vi "Experiment header-Get typedef cluster ref.vi"(8 "error in (no error)":errorcluster, 11 "Header file type":T12) -> (0 "error out":errorcluster, 3 "Header prameter control refs[]":refnum<vi>[](array[refnum]))   [LabVIEW 2013]
uses:
  Typedefs/Header params-Funct acq w rectangles.ctl
  Typedefs/Frame Size.ctl
  Typedefs/Header parameters cluster-Zstack.ctl
  Typedefs/Header parameters cluster-Live imaging.ctl
  Typedefs/AOL modes.ctl
  Typedefs/Plane Mode.ctl
  Typedefs/Header parameters cluster-ALL.ctl
  Typedefs/Imaging Protocols enum.ctl
  Typedefs/Objective selector control enum.ctl
  Typedefs/Header file type enum.ctl
  Typedefs/Controls/AOL_Globals.ctl
panel:
  in  "Parameters tab":T1(tab)
  in  "All header parameters":T2={"Imaging Protocol"=enum."AOL Z-Stack", "Number of POI"=0, "Number of Miniscans"=0, "Number of Trials"=0, "Number of Cycles "=0, "# Averaged Frames"=0, "Laser power (%)"=0, "Pockels"=0.0, "Acquisition Length (sec)"=0.0, "Fill time (us)"=0.0, "POI Dwell time (us)"=0.0, "Miniscan Dwell time per pixel (us)"=0.0, "PMT 1"=0.0, "PMT 2"=0.0, "Back Apperture"=0.0, "Zoom"=0.0, "Frame Size"=0, "Center Frequency"=0.0, "Field of View"=0.0, "DwellTime (us)"=0.0, "Wavelength (nm)"=0.0, "AOL Z"=0.0, "AOL Mode"=enum."Raster", "GridXY"=0.0, "GridZ"=0.0, "TriggerDelay (sec)"=0.0, "Number of Pixels in Miniscan"=0, "Experiment folder path"=path "", "X centre"=0.0, "Y centre"=0.0, "Angle (degrees)"=0.0, "Plane Mode"=0, "Software version"=0.0, "Objective"="Olympus  20X", "MotorZ Calibration"=0, "Pockels Calibration"=0, "Threshold"=[], "Video length (sec)"=0.0, "Frame rate (fps)"=0, "Rectangle ROI length (pixels)"=0, "Rectangle ROI height (pixels)"=0} {"Pockels" format="%#.6g"; "Software version" format="%#.6g"; "Plane Mode" items=["XY Plane"]; "Angle (degrees)" format="%#.6g"; "Frame Size" items=["100X100"=100, "128X128"=128, "200X200"=200, "256X256"=256, "512X512"=512, "1024x1024"=1024, "2048x2048"=2048]; "Back Apperture" format="%#.6g"; "PMT 2" format="%#.6g"; "PMT 1" format="%#.6g"; "Miniscan Dwell time per pixel (us)" format="%#.6g"; "Zoom" format="%#.6g"; "POI Dwell time (us)" format="%#.6g"; "Acquisition Length (sec)" format="%#.6g"; "Fill time (us)" format="%#.6g"}
  in  "Header parameters-Zstack":T8={"Number of POI"=0, "Number of Miniscans"=0, "Number of Trials"=0, "Number of Cycles "=0, "# Averaged Frames"=0, "Laser power (%)"=0, "Pockels"=0.0, "Acquisition Length (sec)"=0.0, "Fill time (us)"=0.0, "DwellTime (us)"=0.0, "Miniscan Dwell time per pixel (us)"=0.0, "PMT 1"=0.0, "PMT 2"=0.0, "Back Apperture"=0.0, "Zoom"=0.0, "Number of Pixels in Miniscan"=0, "Frame Size"=200, "Field of View"=0.0, "X centre"=0.0, "Y centre"=0.0, "AOL Z"=0.0} {"Frame Size" items=["100X100"=100, "128X128"=128, "200X200"=200, "256X256"=256, "512X512"=512, "1024x1024"=1024, "2048x2048"=2048]; "Back Apperture" format="%#.6g"; "Pockels" format="%#.6g"; "PMT 2" format="%#.6g"; "PMT 1" format="%#.6g"; "Miniscan Dwell time per pixel (us)" format="%#.6g"; "Zoom" format="%#.6g"; "DwellTime (us)" format="%#.6g"; "Acquisition Length (sec)" format="%#.6g"; "Fill time (us)" format="%#.6g"}
  in  "Header params-Funct acq w rectangles":T9={"Number of POI"=0, "Number of Miniscans"=0, "Number of Trials"=0, "Number of Cycles "=0, "# Averaged Frames"=0, "Laser power (%)"=0, "Pockels"=0.0, "Acquisition Length (sec)"=0.0, "Fill time (us)"=0.0, "DwellTime (us)"=0.0, "Miniscan Dwell time per pixel (us)"=0.0, "PMT 1"=0.0, "PMT 2"=0.0, "Back Apperture"=0.0, "Zoom"=0.0, "Number of Pixels in Miniscan"=0, "Frame Size"=200, "Field of View"=0.0, "X centre"=0.0, "Y centre"=0.0, "AOL Z"=0.0, "Rectangle ROI length (pixels)"=0, "Rectangle ROI height (pixels)"=0} {"Frame Size" items=["100X100"=100, "128X128"=128, "200X200"=200, "256X256"=256, "512X512"=512, "1024x1024"=1024, "2048x2048"=2048]; "Back Apperture" format="%#.6g"; "Pockels" format="%#.6g"; "PMT 2" format="%#.6g"; "PMT 1" format="%#.6g"; "Miniscan Dwell time per pixel (us)" format="%#.6g"; "Zoom" format="%#.6g"; "DwellTime (us)" format="%#.6g"; "Acquisition Length (sec)" format="%#.6g"; "Fill time (us)" format="%#.6g"}
  in  "Header parameters-Live imaging":T10={"Frame Size"=200, "Field of View"=0.0, "Zoom"=0, "X centre"=0.0, "Y centre"=0.0, "DwellTime (us)"=0.0, "AOL Z"=0.0, "Wavelength (nm)"=0.0, "Laser power (%)"=0, "Pockels"=0.0, "Back Apperture"=0.0, "PMT 1"=0.0, "PMT 2"=0.0, "# Averaged Frames"=0, "AOL Mode"=enum."Raster", "Angle (degrees)"=0.0, "Plane Mode"=0, "Video length (sec)"=0.0, "Frame rate (fps)"=0, "Fill time (us)"=0.0} {"Fill time (us)" format="%#.6g"; "Back Apperture" format="%#.6g"; "Pockels" format="%#.6g"; "Plane Mode" items=["XY Plane"]; "Angle (degrees)" format="%#.6g"; "Frame Size" items=["100X100"=100, "128X128"=128, "200X200"=200, "256X256"=256, "512X512"=512, "1024x1024"=1024, "2048x2048"=2048]; "PMT 2" format="%#.6g"; "PMT 1" format="%#.6g"}
  in  "AOL_Globals":T11={"Imaging Protocol"=enum."AOL Z-Stack", "Number of POI"=0, "Number of Miniscans"=0, "Number of Trials"=0, "Number of Cycles "=0, "# Averaged Frames"=0, "Laser power (%)"=0, "Pockels"=0.0, "Acquisition Length (sec)"=0.0, "Fill time (us)"=0.0, "POI Dwell time (us)"=0.0, "Miniscan Dwell time per pixel (us)"=0.0, "PMT 1"=0.0, "PMT 2"=0.0, "Back Apperture"=200.0, "Frame Size"=0, "Center Frequency"=0.0, "Field of View"=0.0, "DwellTime (us)"=0.0, "Wavelength (nm)"=0.0, "Zoom"=0.0, "AOL Z"=0.0, "AOL Mode"=enum."Raster", "GridXY"=0.0, "GridZ"=0.0, "TriggerPeriod (sec)"=0.0, "Number of Pixels in Miniscan"=0, "Experiment folder path"=path "", "X centre"=0.0, "Y centre"=0.0, "Angle (degrees)"=0.0, "Plane Mode"=0, "Threshold"=[], "Regenerate Chirps"=FALSE, "Rectangle ROI length (pixels)"=0, "Rectangle ROI height (pixels)"=0, "AOD fill"=0, "Samples Wait after Trigger"=0, "StartUp Delay"=0, "Slip Cycle"=163840, "Add Cycle"=FALSE} {"Plane Mode" items=["XY Plane"]; "Frame Size" items=["100X100"=100, "128X128"=128, "200X200"=200, "256X256"=256, "512X512"=512, "1024x1024"=1024, "2048x2048"=2048]; "Back Apperture" format="%#.6g"; "Pockels" format="%#.6g"; "PMT 2" format="%#.6g"; "PMT 1" format="%#.6g"; "Angle (degrees)" format="%#.6g"; "POI Dwell time (us)" format="%#.6g"}
  # "Zstack header parameters"
  # "Zstack header parameters"
  # "Live imaging header parameters"
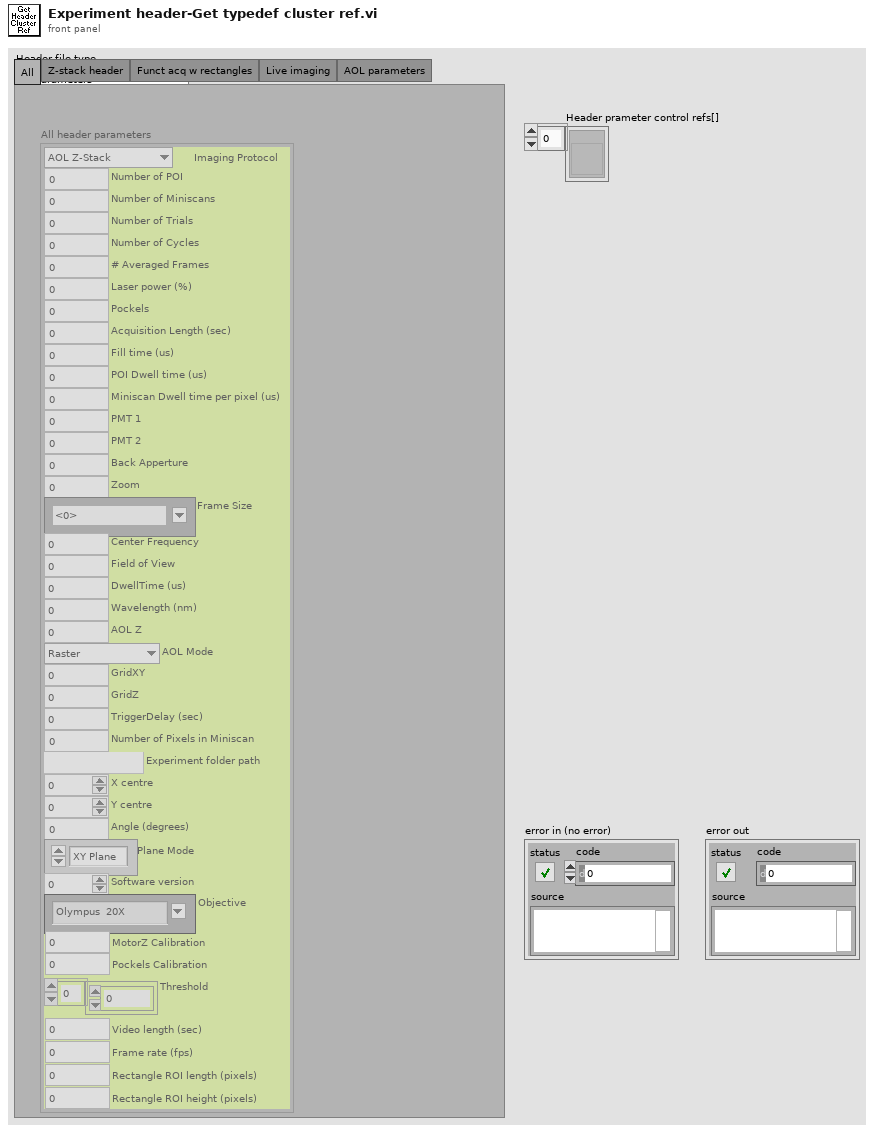
[diagram p1: front panel]
types:
  T1 = enum32{"All", "Z-stack header", "Funct acq w rectangles", "Live imaging", "AOL parameters"}
  T2 = typedef "Header parameters cluster-ALL.ctl" = cluster{"Imaging Protocol":T3, "Number of POI":u16, "Number of Miniscans":u16, "Number of Trials":u16, "Number of Cycles ":u64, "# Averaged Frames":u16, "Laser power (%)":u8, "Pockels":dbl, "Acquisition Length (sec)":dbl, "Fill time (us)":dbl, "POI Dwell time (us)":dbl, "Miniscan Dwell time per pixel (us)":dbl, "PMT 1":dbl, "PMT 2":dbl, "Back Apperture":dbl, "Zoom":dbl, "Frame Size":T4, "Center Frequency":dbl, "Field of View":dbl, "DwellTime (us)":dbl, "Wavelength (nm)":dbl, "AOL Z":dbl, "AOL Mode":T5, "GridXY":dbl, "GridZ":dbl, "TriggerDelay (sec)":dbl, "Number of Pixels in Miniscan":u16, "Experiment folder path":path, "X centre":dbl, "Y centre":dbl, "Angle (degrees)":dbl, "Plane Mode":T6, "Software version":dbl, "Objective":T7, "MotorZ Calibration":u32, "Pockels Calibration":u32, "Threshold":u16[], "Video length (sec)":dbl, "Frame rate (fps)":u8, "Rectangle ROI length (pixels)":u16, "Rectangle ROI height (pixels)":u16}
  T3 = typedef "Imaging Protocols enum.ctl" = enum16{"AOL Z-Stack", "Motor Z Stack", "Functional Acquisition", "Single Plane Acquisition", "Volume Acquisition", "Live Imaging", "Live Plane Imaging", "Live Volume Imaging"}
  T4 = typedef "Frame Size.ctl" = u16
  T5 = typedef "AOL modes.ctl" = enum16{"Raster", "Structural", "Pointing", "Mini Scan", "Alignment"}
  T6 = typedef "Plane Mode.ctl" = u16
  T7 = typedef "Objective selector control enum.ctl" = string
  T8 = typedef "Header parameters cluster-Zstack.ctl" = cluster{"Number of POI":u16, "Number of Miniscans":u16, "Number of Trials":u16, "Number of Cycles ":u16, "# Averaged Frames":u16, "Laser power (%)":u8, "Pockels":dbl, "Acquisition Length (sec)":dbl, "Fill time (us)":dbl, "DwellTime (us)":dbl, "Miniscan Dwell time per pixel (us)":dbl, "PMT 1":dbl, "PMT 2":dbl, "Back Apperture":dbl, "Zoom":dbl, "Number of Pixels in Miniscan":u16, "Frame Size":T4, "Field of View":dbl, "X centre":dbl, "Y centre":dbl, "AOL Z":dbl}
  T9 = typedef "Header params-Funct acq w rectangles.ctl" = cluster{"Number of POI":u16, "Number of Miniscans":u16, "Number of Trials":u16, "Number of Cycles ":u16, "# Averaged Frames":u16, "Laser power (%)":u8, "Pockels":dbl, "Acquisition Length (sec)":dbl, "Fill time (us)":dbl, "DwellTime (us)":dbl, "Miniscan Dwell time per pixel (us)":dbl, "PMT 1":dbl, "PMT 2":dbl, "Back Apperture":dbl, "Zoom":dbl, "Number of Pixels in Miniscan":u16, "Frame Size":T4, "Field of View":dbl, "X centre":dbl, "Y centre":dbl, "AOL Z":dbl, "Rectangle ROI length (pixels)":u16, "Rectangle ROI height (pixels)":u16}
  T10 = typedef "Header parameters cluster-Live imaging.ctl" = cluster{"Frame Size":T4, "Field of View":dbl, "Zoom":u16, "X centre":dbl, "Y centre":dbl, "DwellTime (us)":dbl, "AOL Z":dbl, "Wavelength (nm)":dbl, "Laser power (%)":u8, "Pockels":dbl, "Back Apperture":dbl, "PMT 1":dbl, "PMT 2":dbl, "# Averaged Frames":u8, "AOL Mode":T5, "Angle (degrees)":dbl, "Plane Mode":T6, "Video length (sec)":dbl, "Frame rate (fps)":u8, "Fill time (us)":dbl}
  T11 = typedef "AOL_Globals.ctl" = cluster{"Imaging Protocol":T3, "Number of POI":u16, "Number of Miniscans":u16, "Number of Trials":u16, "Number of Cycles ":u64, "# Averaged Frames":u16, "Laser power (%)":u8, "Pockels":dbl, "Acquisition Length (sec)":dbl, "Fill time (us)":dbl, "POI Dwell time (us)":dbl, "Miniscan Dwell time per pixel (us)":dbl, "PMT 1":dbl, "PMT 2":dbl, "Back Apperture":dbl, "Frame Size":T4, "Center Frequency":dbl, "Field of View":dbl, "DwellTime (us)":dbl, "Wavelength (nm)":dbl, "Zoom":dbl, "AOL Z":dbl, "AOL Mode":T5, "GridXY":dbl, "GridZ":dbl, "TriggerPeriod (sec)":dbl, "Number of Pixels in Miniscan":u16, "Experiment folder path":path, "X centre":dbl, "Y centre":dbl, "Angle (degrees)":dbl, "Plane Mode":T6, "Threshold":u16[], "Regenerate Chirps":bool, "Rectangle ROI length (pixels)":u16, "Rectangle ROI height (pixels)":u16, "AOD fill":u16, "Samples Wait after Trigger":u16, "StartUp Delay":i32, "Slip Cycle":u32, "Add Cycle":bool}
  T12 = typedef "Header file type enum.ctl" = enum16{"All parameters", "Params for funct acq w ROI or mscn", "Params for funct acq w rectangles", "Live imaging header parameters", "AOL Parameters"}
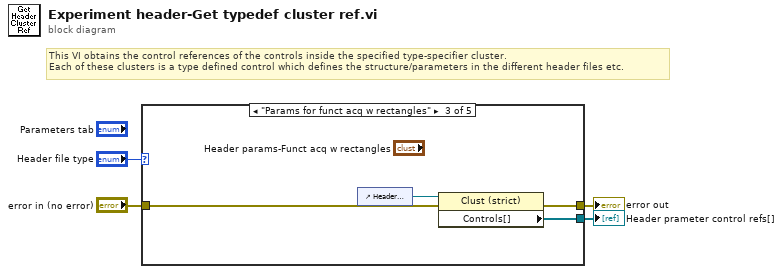
[diagram p0: block diagram]
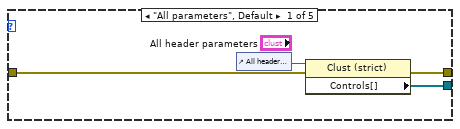
[diagram p2: hidden frame]
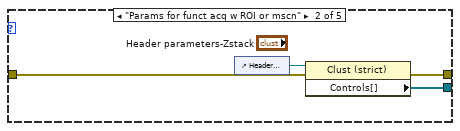
[diagram p3: hidden frame]
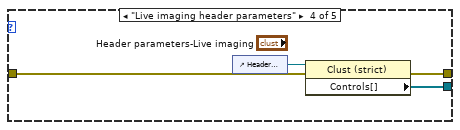
[diagram p4: hidden frame]
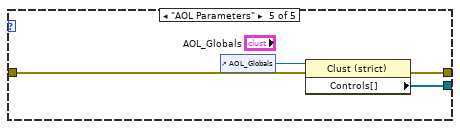
[diagram p5: hidden frame]
diagram:
  # "This VI obtains the control references of the controls inside the specified type-specifier cluster.\nEach of these clusters is a type defined control which defines the structure/parameters in the different header files etc."
  n1 = case shown="\"Params for funct acq w rectangles\"" "Header file type" {
    tunnel: [w8 w11 w16 w18 w22] -> w3
    tunnel: "error in (no error)" -> [w7 w10 w15 w17 w21]
    tunnel: [w6 w9 w14 w19 w23] -> w1
    frame "All parameters", Default {
      n2 = control-ref of="All header parameters"() -> (w5:refnum<vi>)
      n3 = property on="Property Node" class="Clust (strict)"(reference=w5, error in=w7) -> (error out=w6:errorcluster, "Controls[]"=w8:refnum<vi>[])  [unwired: 1 out]
    }
    frame "Params for funct acq w ROI or mscn" {
      n4 = control-ref of="Header parameters-Zstack"() -> (w12:refnum<vi>)
      n5 = property on="Property Node" class="Clust (strict)"(reference=w12, error in=w10) -> (error out=w9:errorcluster, "Controls[]"=w11:refnum<vi>[])  [unwired: 1 out]
    }
    frame "Params for funct acq w rectangles" {
      n6 = control-ref of="Header params-Funct acq w rectangles"() -> (w13:refnum<vi>)
      n7 = property on="Property Node" class="Clust (strict)"(reference=w13, error in=w15) -> (error out=w14:errorcluster, "Controls[]"=w16:refnum<vi>[])  [unwired: 1 out]
    }
    frame "Live imaging header parameters" {
      n8 = control-ref of="Header parameters-Live imaging"() -> (w20:refnum<vi>)
      n9 = property on="Property Node" class="Clust (strict)"(reference=w20, error in=w17) -> (error out=w19:errorcluster, "Controls[]"=w18:refnum<vi>[])  [unwired: 1 out]
    }
    frame "AOL Parameters" {
      n10 = control-ref of="AOL_Globals"() -> (w24:refnum<vi>)
      n11 = property on="Property Node" class="Clust (strict)"(reference=w24, error in=w21) -> (error out=w23:errorcluster, "Controls[]"=w22:refnum<vi>[])  [unwired: 1 out]
    }
  }
  "Header prameter control refs[]" <- w3
  "error out" <- w1
